vi "Constants.vi"() -> ()   [LabVIEW 2017]
uses:
  TypeDef_PIDFgains.ctl
  <vilib>/Rock Robotics/WPI/ThirdParty/Phoenix-LabVIEW/Motor Controller/Controls/CTRE_Phoenix_MotorControl_RemoteSourceType.ctl
  <vilib>/Rock Robotics/WPI/ThirdParty/Phoenix-LabVIEW/Motor Controller/Controls/CTRE_Phoenix_MotorControl_SensorTermFeedbackDevice_Enhanced.ctl
  <vilib>/Rock Robotics/WPI/Solenoid/WPI_SolenoidChannel.ctl
panel:
  in  "Solenoid Channel":cluster{"Low gear":T1, "High gear":T1}
  in  "Remote 0":cluster{"Remote Device Type":T2, "Slot name":T3} {"Slot name" items=["None"=-1, "QuadEncoder"=0, "Analog"=2, "Tachometer"=4, "Pulse Width Encoded Position"=8, "Remote Source 0"=11, "Remote Source 1"=12, "Software Emulated"=15]}
  in  "sensor phase right":bool
  in  "sensor phase left":bool
  in  "invert right":bool
  in  "invert left":bool=TRUE
  in  "CAN  IDs":T4={"left talon"=1, "left victor 0"=2, "left victor 1"=3, "right talon"=4, "right victor 0"=5, "right victor 1"=6, "pigeon"=-5}
  in  "PIDF Aux":i32=1
  in  "PIDF Primary":i32
  in  "Turn Travel\nUnits Per Rotation":dbl=3600.0
  in  "high turn PIDF":T5={"kP"=0.3, "kI "=0.0, "kD"=0.0, "kF"=0.02692105263, "I Zone"=0.0, "Peak Out"=1.0}
  in  "high PIDF":T5={"kP"=0.15, "kI "=0.0, "kD"=0.0, "kF"=0.01346052631, "I Zone"=0.0, "Peak Out"=1.0}
  in  "low turn PIDF":T5={"kP"=0.08, "kI "=0.0, "kD"=0.0, "kF"=0.05683333333, "I Zone"=0.0, "Peak Out"=1.0}
  in  "low PIDF":T5={"kP"=0.04, "kI "=0.0, "kD"=0.0, "kF"=0.02841666666, "I Zone"=0.0, "Peak Out"=1.0}
  in  "Timeout Ms":i32=10
  in  "Pigeon Units\nPer Rotatoin":i32=8192
  in  "Sensor Units\nPer Rotation":i32=4096
  in  "high turn slot":i32=3
  in  "high velocity slot":i32=2
  in  "low turn slot":i32=1
  in  "low velocity slot":i32
  # "Scales units to\n3600 per rotation.\nThis is nice, as it\nmeans one unit is\n0.1 degrees."
  # "How many\nsensor units\nper rotation:\nCTRE Mag\nEncoder"
  # "Property of pigeon\nshould not be\nchanged"
  # "0 - Skip confirmation\nNonZero - Wait and log\nto DS if something fails"
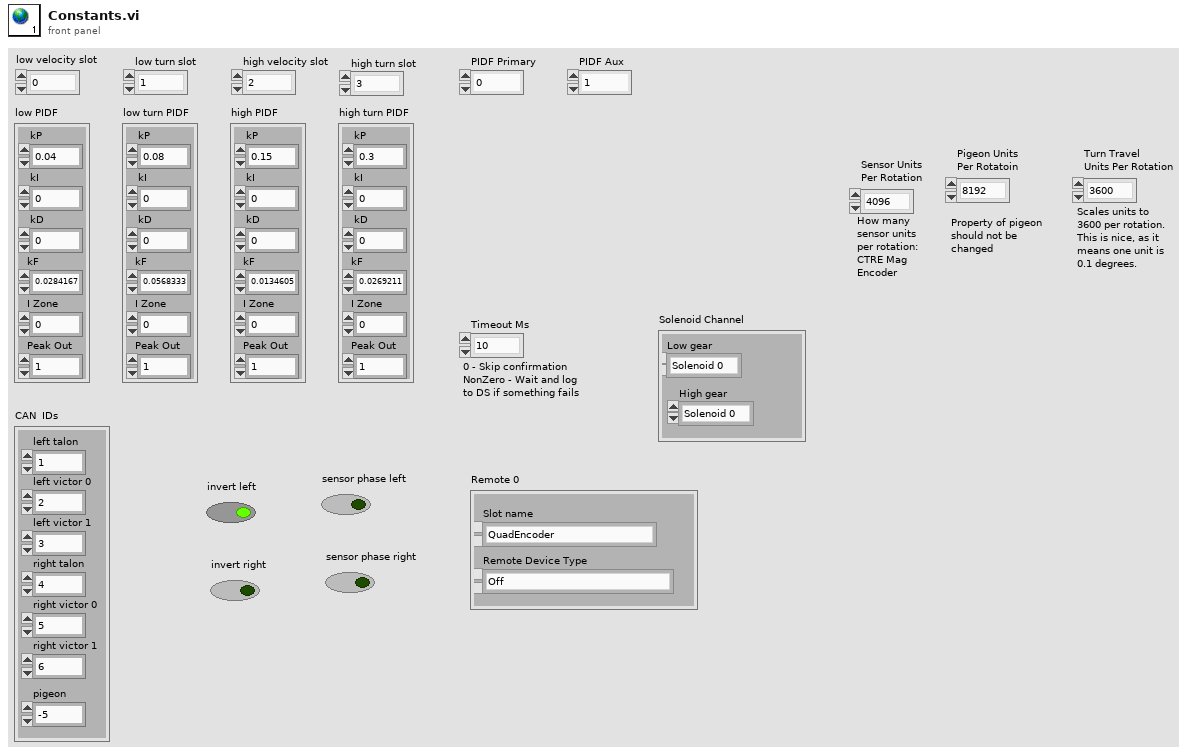
[diagram p1: front panel]
types:
  T1 = typedef "WPI_SolenoidChannel.ctl" = enum8{"Solenoid 0", "Solenoid 1", "Solenoid 2", "Solenoid 3", "Solenoid 4", "Solenoid 5", "Solenoid 6", "Solenoid 7", "Invalid"}
  T2 = typedef "CTRE_Phoenix_MotorControl_RemoteSourceType.ctl" = enum16{"Off", "Talon SRX Selected Sensor", "Pigeon IMU Yaw", "Pigeon IMU Pitch", "Pigeon IMU Roll", "CANifier Quadrature", "CANifier PWM Input 0", "CANifier PWM Input 1", "CANifier PWM Input 2", "CANifier PWM Input 3", "Gadgeteer Pigeon Yaw", "Gadgeteer Pigeon Pitch", "Gadgeteer Pigeon Roll"}
  T3 = typedef "CTRE_Phoenix_MotorControl_SensorTermFeedbackDevice_Enhanced.ctl" = i8
  T4 = cluster{"left talon":i32, "left victor 0":i32, "left victor 1":i32, "right talon":i32, "right victor 0":i32, "right victor 1":i32, "pigeon":i32}
  T5 = typedef "TypeDef_PIDFgains.ctl" = cluster{"kP":dbl, "kI ":dbl, "kD":dbl, "kF":dbl, "I Zone":dbl, "Peak Out":dbl}
diagram:
